vi "Add Protection.vi"(8 "error in (no error)":errorcluster, 9 "Pad":bool, 10 "String in":string, 11 "CRC-32 in":refnum<class "CRC-32.lvclass">) -> (0 "error out":errorcluster, 2 "String out":string, 3 "CRC-32 out":refnum<class "CRC-32.lvclass">)   [LabVIEW 2023, in "Protections.lvlib" / "CRC-32.lvclass"]
uses:
  CRC-32.lvclass
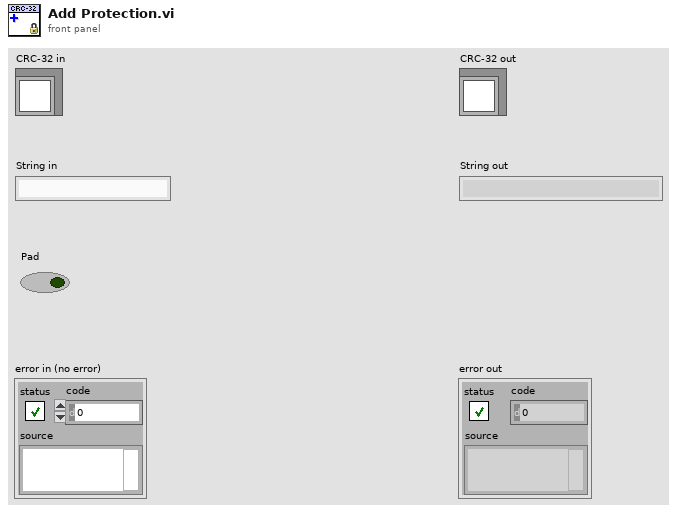
[diagram p1: front panel]
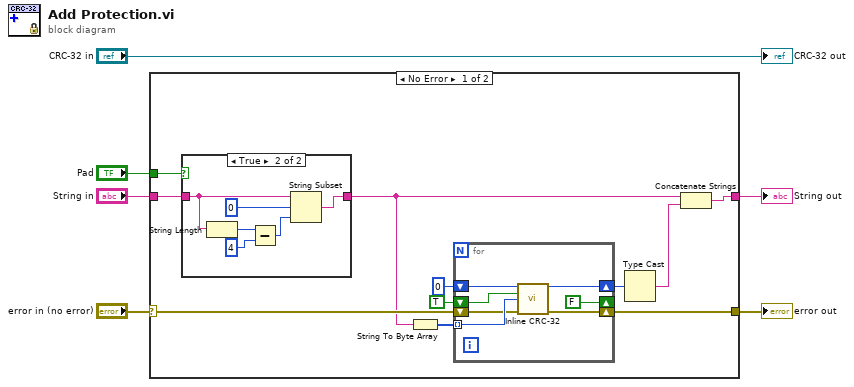
[diagram p0: block diagram]
diagram:
  n1 = case shown="No Error" "error in (no error)" {
    selector: "error in (no error)" -> [w10 w33]
    tunnel: [w17 w32] -> w6
    tunnel: "String in" -> [w9 w32]
    tunnel: "Pad" -> [w8 _]
    tunnel: [w13 w33] -> w2
    frame No Error {
      n2 = case shown="True" w8 {
        tunnel: w9 -> [w18 w24]
        tunnel: [w18 w19] -> w7
        frame False {
        }
        frame True {
          n3 = String Length(string=w24) -> (length=w22:i32)
          n4 = Subtract(x=w22, y=4) -> (x-y=w20:i32)
          n5 = String Subset(string=w24, offset (0)=0, length (rest)=w20) -> (substring=w19:string)
        }
      }
      n6 = String To Byte Array(string=w7) -> (unsigned byte array=w15:u8[])
      n7 = for {
        shift-right: [w30] -> w12
        shift-left: u32 0 ("CRC") -> [w31]
        tunnel: w15 -> [w29] mode=indexing
        shift-right: [w27] -> w13
        shift-left: w10 -> [w28]
        shift-right: [FALSE] -> _
        shift-left: TRUE -> [w26]
        n8 = call "Inline CRC-32.vi"("CRC In"=w31, "Reset"=w26, "Data"=w29, "error in (no error)"=w28) -> ("CRC"=w30:u32, "error out"=w27:errorcluster)  [unwired: 10 in]
      }
      n9 = Type Cast(x=w12) -> (*(type *) &x=w11:string)  [unwired: 1 in]
      n10 = Concatenate Strings(w7, w11) -> (w17:string)
    }
    frame Error {
    }
  }
  "error out" <- w2
  "String out" <- w6
  "CRC-32 out" <- "CRC-32 in"
